vi "PID.vi"(0 "Sensor Input":dbl, 2 "Setpoint":dbl, 3 "Kp":dbl=1.0, 5 "Ki":dbl=0.3, 8 "Prev Time":dbl, 9 "Kd":dbl=0.2, 10 "Curr Time":dbl, 11 "Accumulate In":dbl, 16 "Previous Error":dbl) -> (7 "Kp Gain":dbl, 13 "Ki Gain":dbl, 14 "Output Val":dbl, 17 "Accumulate Out":dbl, 18 "Kd gain":dbl, 19 "Current Error":dbl)   [LabVIEW 2016]
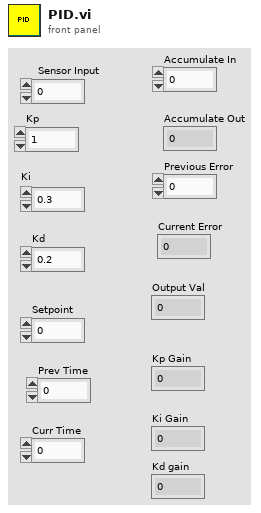
[diagram p1: front panel]
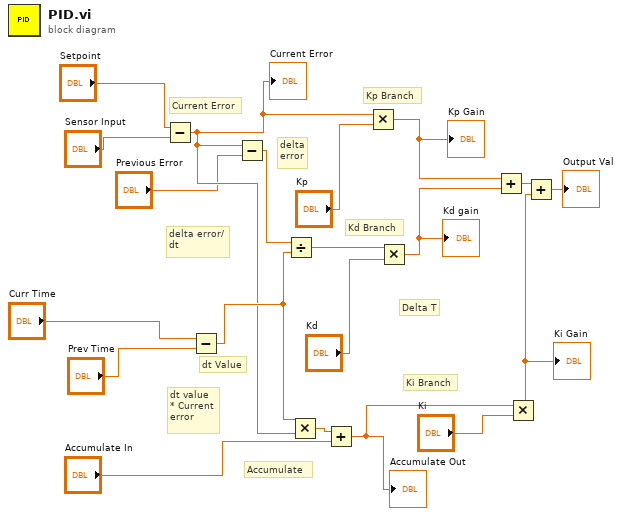
[diagram p0: block diagram]
diagram:
  # "Delta T"
  # "Accumulate"
  # "dt value\n* Current\nerror"
  # "delta error/\ndt"
  # "delta\nerror"
  # "dt Value"
  # "Current Error"
  # "Ki Branch"
  # "Kd Branch"
  # "Kp Branch"
  n1 = Subtract(x="Setpoint", y="Sensor Input") -> (x-y=w9:dbl)
  "Current Error" <- w9
  n2 = Subtract(x="Curr Time", y="Prev Time") -> (x-y=w12:dbl)
  n3 = Subtract(x=w9, y="Previous Error") -> (x-y=w13:dbl)
  n4 = Divide(x=w13, y=w12) -> (x/y=w17:dbl)
  n5 = Multiply(x=w12, y=w9) -> (x*y=w15:dbl)
  n6 = Add(x=w15, y="Accumulate In") -> (x+y=w4:dbl)
  "Accumulate Out" <- w4
  n7 = Multiply(x=w9, y="Kp") -> (x*y=w2:dbl)
  "Kp Gain" <- w2
  n8 = Multiply(x=w17, y="Kd") -> (x*y=w3:dbl)
  "Kd gain" <- w3
  n9 = Add(x=w2, y=w3) -> (x+y=w19:dbl)
  n10 = Multiply(x=w4, y="Ki") -> (x*y=w1:dbl)
  "Ki Gain" <- w1
  n11 = Add(x=w19, y=w1) -> (x+y=→"Output Val":dbl)
